vi "DialogCreateInterface.vi"(0 "ClassWriterNative.lvclass":refnum<class "ClassWriterNative.lvclass">, 1 "ProjectItem Refnum":refnum<vi>, 5 "error in (no error)":errorcluster) -> (14 "Reference out":refnum<class "ClassWriterNative.lvclass">, 15 "Cancelled":bool, 16 "CreateInterfaceData":T3, 19 "error out":errorcluster)   [LabVIEW 2020, in "ClassWriterNative.lvclass"]
uses:
  <resource>/Framework/Providers/Open_GDS/ClassProviders/Provider_LvNativeClass/ClassWriterNative_class/ClassWriterNative.lvclass
  <resource>/Framework/Providers/Open_GDS/ClassProviders/Provider_BaseClassInterface/CreateInterfaceData.ctl
  <resource>/Framework/Providers/Open_GDS/ClassProviders/Provider_BaseClassInterface/ClassWriter_class/InterfaceMethodsToCreate.ctl
  <resource>/Framework/Providers/Open_GDS/ClassProviders/Common/CommonVIs/CommonVIs_AttributeType.ctl
  <resource>/Framework/Providers/Open_GDS/ClassProviders/Common/CommonVIs/CommonVIs_AttributeDataType.ctl
  <resource>/Framework/Providers/Open_GDS/ClassProviders/Common/String/GDSString_AccessScopeModifierType.ctl
  <resource>/Framework/Providers/Open_GDS/ClassProviders/Provider_BaseClassInterface/ClassWriter_class/InterfacesToImplement.ctl
  <resource>/Framework/Providers/Open_GDS/ClassProviders/Provider_BaseClassInterface/BaseProvider_SubVIs/BaseProvider_WireList.ctl
  <resource>/Framework/Providers/Open_GDS/ClassProviders/Provider_BaseClassInterface/BaseProvider_SubVIs/BaseProvider_WireStyleType.ctl
  <vilib>/Utility/miscctls.llb/LVRectTypeDef.ctl
  <resource>/Framework/Providers/Open_GDS/ClassProviders/Common/InterfaceLibrary/InterfaceInfo.ctl
  <resource>/Framework/Providers/Open_GDS/ClassProviders/Common/LvClass_class/GDSLvClass_ClassMethodInfo.ctl
  <resource>/Framework/Providers/Open_GDS/ClassProviders/Common/CommonVIs/CommonVIs_ClassIconSelection_Action.ctl
  <vilib>/Utility/miscctls.llb/LVPositionTypeDef.ctl
  <vilib>/picture/picture.llb/imagedata.ctl
  <vilib>/Utility/miscctls.llb/LVRowAndColumnUnsignedTypeDef.ctl
  8226ef7b-d77c-4b82-be33-8974597c5039.vi
  <resource>/Framework/Providers/Open_GDS/ClassProviders/Common/InterfaceLibrary/InterfaceLibrary.lvlib
  <resource>/Framework/Providers/Open_GDS/ClassProviders/Provider_BaseClassInterface/ClassWriter_class/ClassWriter.lvclass
panel:
  out "IconSelection":picture
  in  "WireSelectionList":T1
  out "Wire Style":cluster{"Name":string, "Wire":picture}
  in  "InterfaceFilter":string caption="Filter"
  out "Icon":picture
  in  "_ShowContextHelp":bool
  in  "Help":bool
  in  "ConnectorPanePattern":u16(ring) caption="Connector Pane" items=["4x4x4", "5x6x5", "6x8x6"]
  in  "_UseLLB":bool
  in  "_InterfaceFolderSuffix":string caption="Interface Folder Suffix"
  out "ProductPicture":picture
  out "DupPath":bool
  in  "_InterfaceName":string caption="Interface Name"
  in  "_ClassDescription":string caption="Interface Description"
  in  "_InterfaceFolder":path caption="Save Interface To.."
  out "TriggerSuffixChange":string
  in  "SelectInterfaceClass":i32[](listbox) caption="Select Parent Interface(s) (ctrl+click to do multiple Selection)"
  in  "Methods":string[][](table) caption="3 methods selected"
  in  "Cancel":bool
  in  "CreateInterface":bool
  # "Icon"
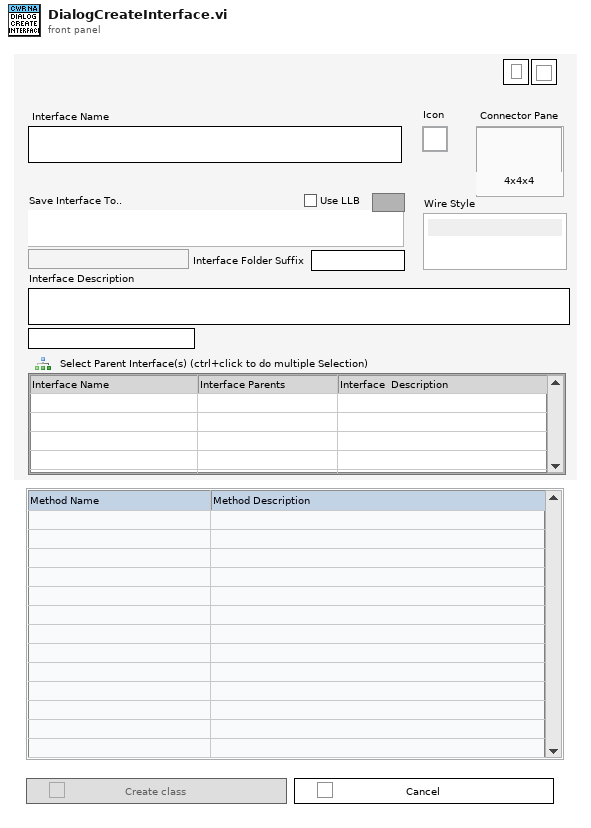
[diagram p1: front panel]
types:
  T1 = typedef "BaseProvider_WireList.ctl" = cluster{"WireStyle":T2[], "WireEditor":bool}
  T2 = typedef "BaseProvider_WireStyleType.ctl" = cluster{"Boolean":bool, "Wire":picture, "Name":string, "Status":u16}
  T3 = typedef "ClassWriter.lvclass/CreateInterfaceData.ctl" = cluster{"InterfaceName":string, "InterfaceFolder":path, "InterfaceDescription":string, "FolderSuffix":string, "MethodsToCreate":T4[], "ParentInterfaces":T8}
  T4 = typedef "ClassWriter.lvclass/InterfaceMethodsToCreate.ctl" = cluster{"Name":string, "Description":string, "MethodsArgumentsIn":T5[], "MethodsArgumentsOut":T5[]}
  T5 = typedef "CommonVIs_AttributeType.ctl" = cluster{"Name":string, "DataType":T6, "ArrayDim":i32, "CtrlPath":path, "DataTypeString":string, "AccessScope":T7, "InitialData":variant}
  T6 = typedef "CommonVIs_AttributeDataType.ctl" = enum16{"UINT8", "INT8", "UINT16", "INT16", "UINT32", "INT32", "UINT64", "INT64", "SGL", "DBL", "EXT", "CSG", "CDB", "CXT", "TimeStamp", "STRING", "PATH", "BOOL", "ENUM", "RefNum", "VIRefNum", "LabVIEW Class", "Cluster", "Variant", "TypeDef", "Waveform", "LabVIEW Object", "Other", "void"}
  T7 = typedef "GDSString_AccessScopeModifierType.ctl" = enum16{"public", "private", "protected", "internal"}
  T8 = typedef "ClassWriter.lvclass/InterfacesToImplement.ctl" = cluster{"InterfacePath":path[], "CreateMethods":bool, "MethodsPerInterface(Empty=>All)":cluster{"Methods":string[]}[]}
  T9 = typedef "LVPositionTypeDef.ctl" = cluster{"Left":i32, "Top":i32}
  T10 = cluster{"Font Name":string, "Size":u16, "Bold":bool, "Italic":bool, "Underline":bool, "Strikeout":bool, "Color":u32}
  T11 = typedef "CommonVIs_ClassIconSelection_Action.ctl" = enum16{"All", "Non Interface", "Only Interface"}
  T12 = typedef "LVRectTypeDef.ctl" = cluster{"Left":i16, "Top":i16, "Right":i16, "Bottom":i16}
  T13 = typedef "InterfaceLibrary.lvlib/InterfaceInfo.ctl" = cluster{"Name(Short if no Conflicts)":string, "FullQualifierName":string, "Description":string, "Path":path, "ParentInterfaceNames(Short if no Conflitcs)":string[], "ParentInterfaceFullQualifierNames":string[], "IconPath":path, "Methods":T14[], "DynamicDispatchMethod":bool[]}
  T14 = typedef "GDSLvClass_ClassMethodInfo.ctl" = cluster{"Name":string, "Descriptions":string, "RelativePath":path, "SourceScope":enum32{"invalid scope", "public", "private", "protected", "community"}, "MustOverride":bool, "VirtualFolderLocation":string[]}
  T15 = cluster{"Cancel":bool, "Derived":bool, "DeriveFromClassRef":refnum<vi>, "ClassPaths":path[], "DesignPatternsVisible":bool, "ClassProviderName":string, "InitDerived":bool, "ClassFolderSuffix":string, "LLB_Allowed":bool, "StartFolder":path, "SplitterMouseDown":bool, "OldBnds":T12, "BondsChanged":bool, "StartBnds":T12, "InterfaceInfo":T13[], "InterfaceIcons":path[]}
  T16 = typedef "LVPointTypeDef.ctl" = cluster{"Horizontal":i16, "Vertical":i16}
  T17 = enum8{"Enabled", "Disabled", "Disabled and Grayed Out"}
  T18 = typedef "imagedata.ctl" = cluster{"image type":i32, "image depth":i32, "image":u8[], "mask":u8[], "colors":u32[], "Rectangle":cluster{"left":i16, "top":i16, "right":i16, "bottom":i16}}
  T19 = typedef "LVRowAndColumnUnsignedTypeDef.ctl" = cluster{"Row":u32, "Column":u32}
  T20 = typedef "BaseProvider_IniFileSettings.ctl" = cluster{"ClassFolderSuffix":string, "InterfaceFolderSuffix":string, "InterfaceIcon":string}
  T21 = typedef "Scripting_ConnectorPanePatternType.ctl" = u16
  T22 = enum32{"Invalid", "Standard", "Closed", "Hidden", "Minimized", "Maximized"}
  T23 = typedef "GOOP_WireConfigurationType.ctl" = cluster{"Edge thickness":i32, "Edge color":u32, "Center thickness":i32, "Center pattern":T24, "CenterColor1":u32, "CenterColor2":u32, "Tunnels and terminals colors":u32}
  T24 = typedef "GOOP_WirePattern.ctl" = enum16{"Solid", "Large dash", "Small dash"}
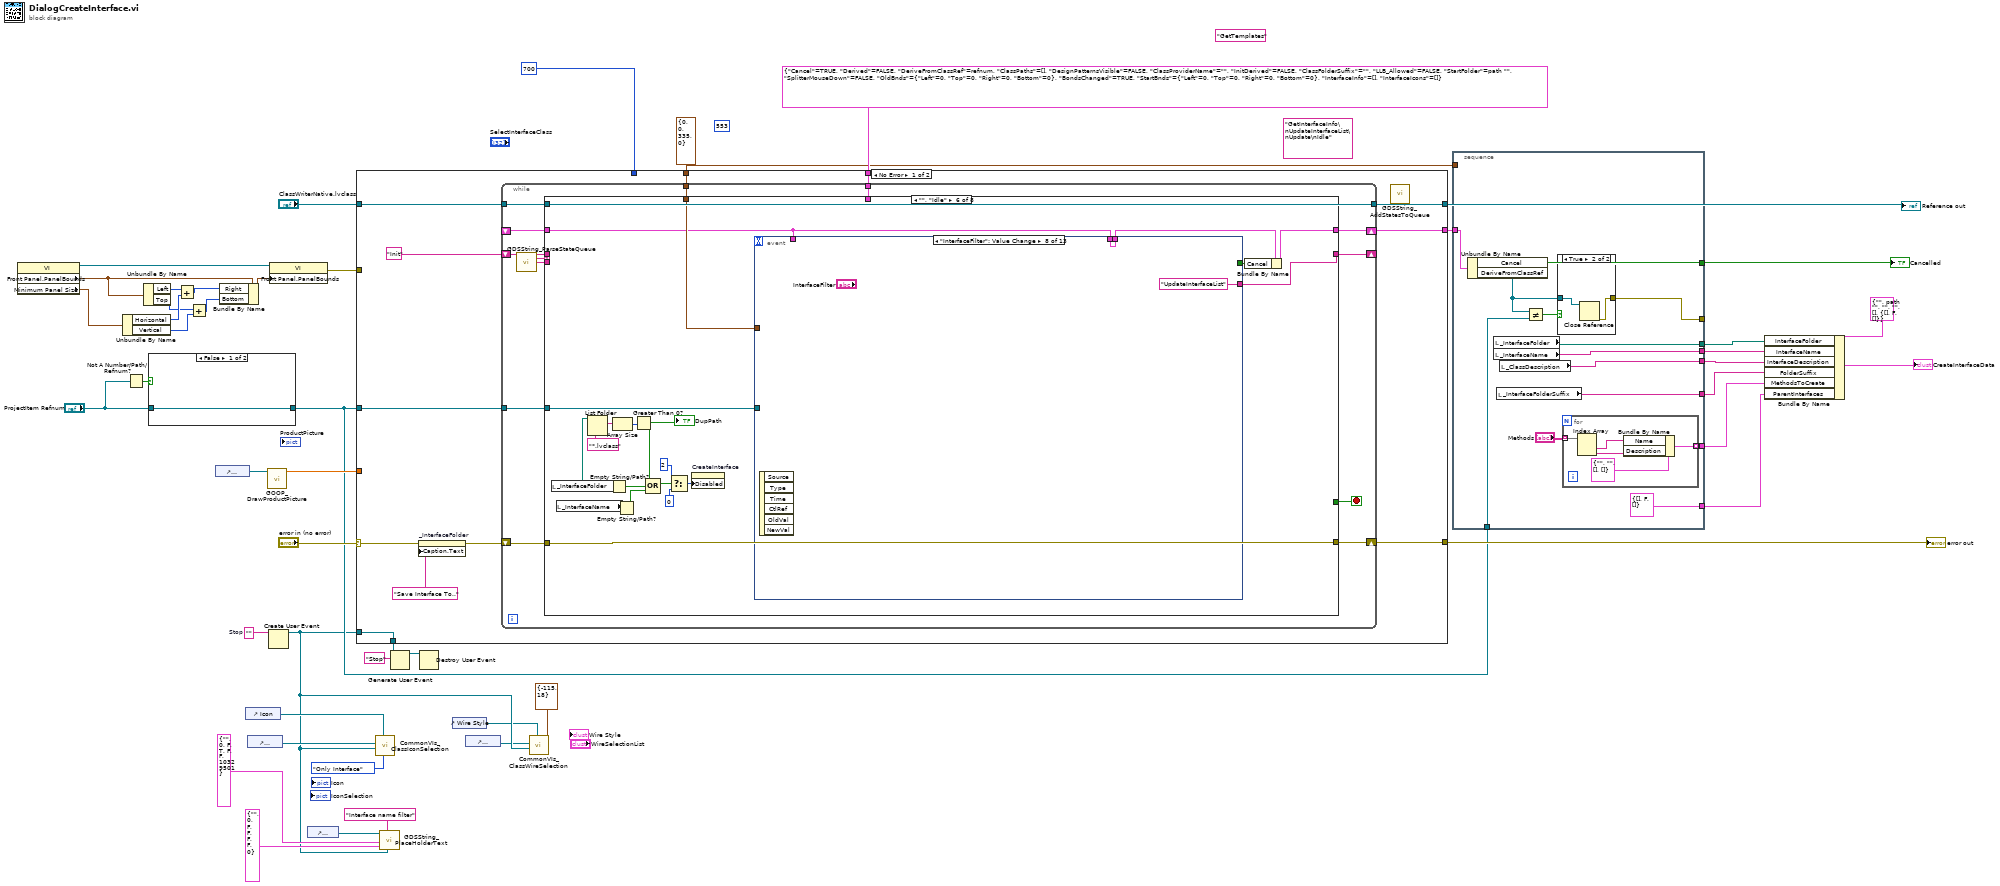
[diagram p0: block diagram]
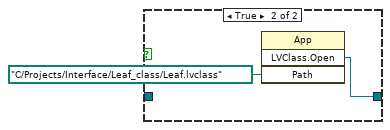
[diagram p2: hidden frame]
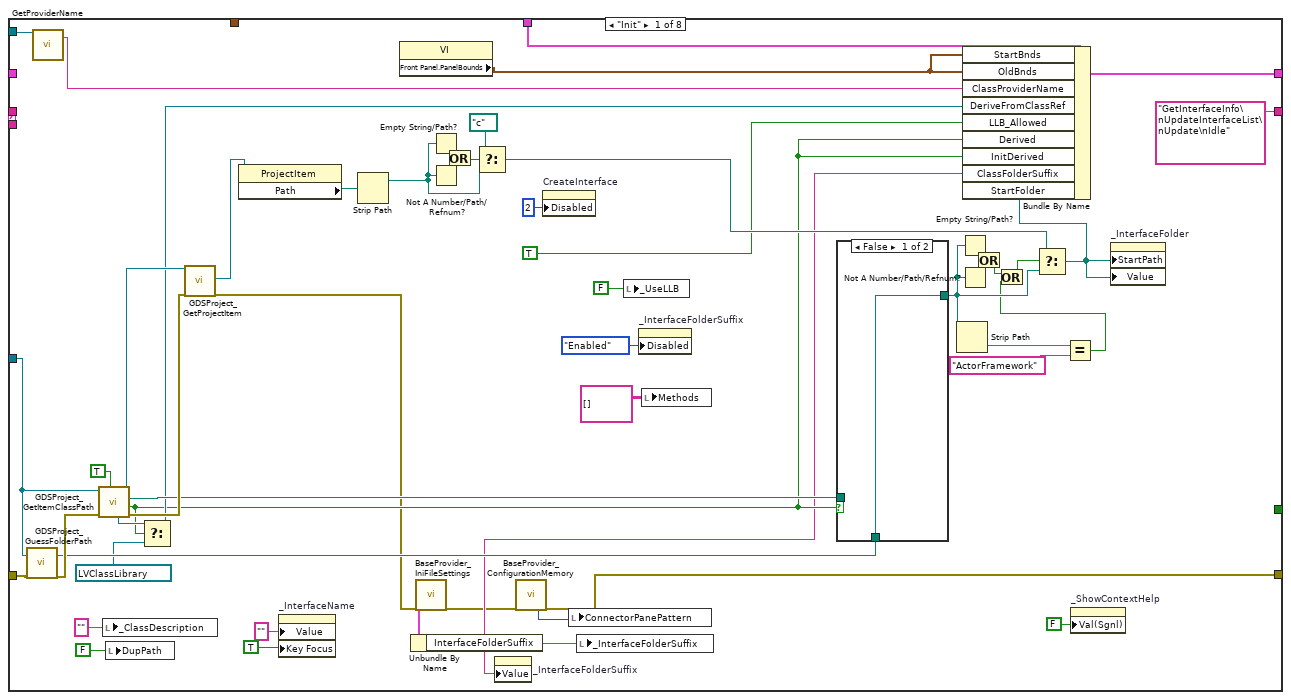
[diagram p4: hidden frame]
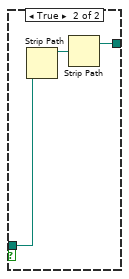
[diagram p5: hidden frame]
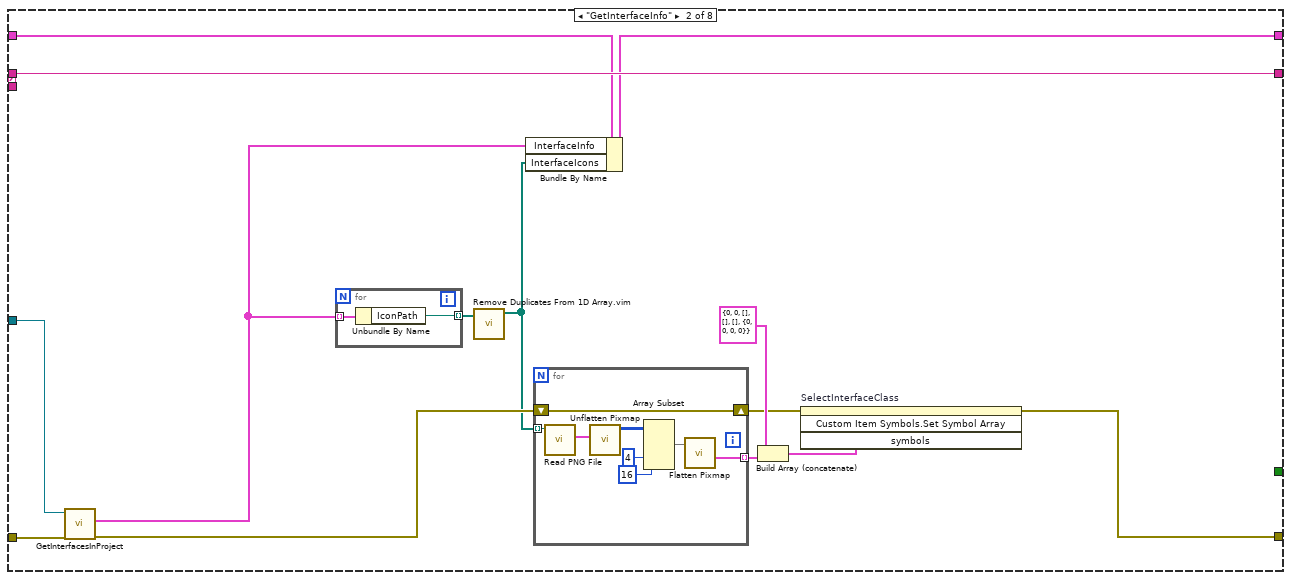
[diagram p6: hidden frame]
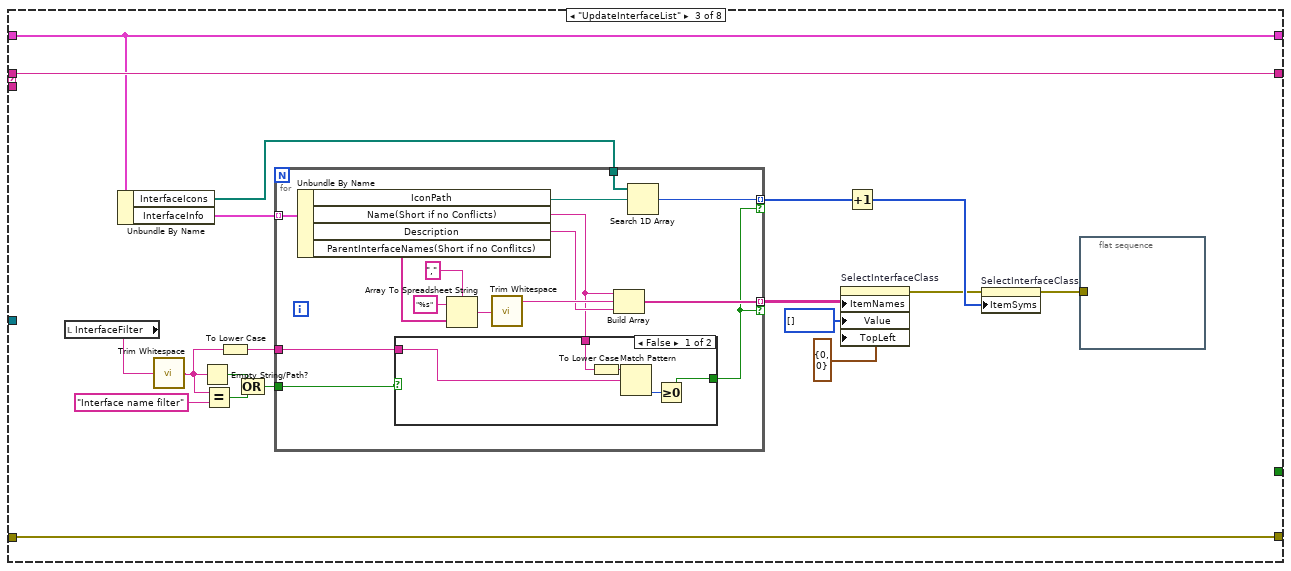
[diagram p7: hidden frame]
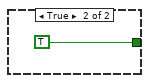
[diagram p8: hidden frame]
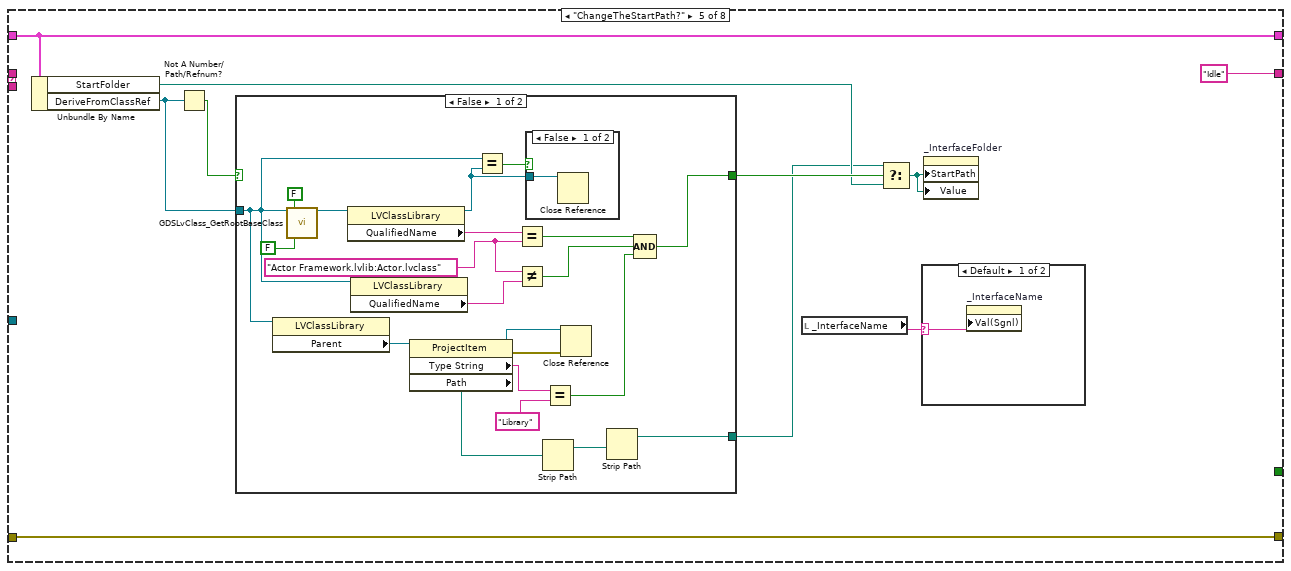
[diagram p10: hidden frame]
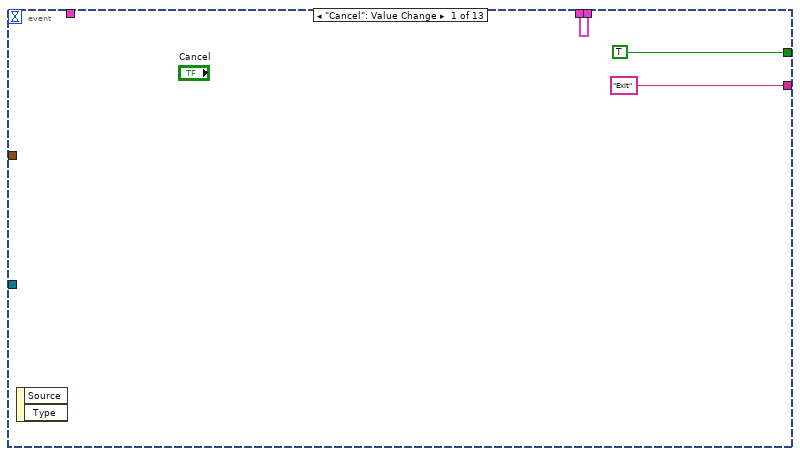
[diagram p14: hidden frame]
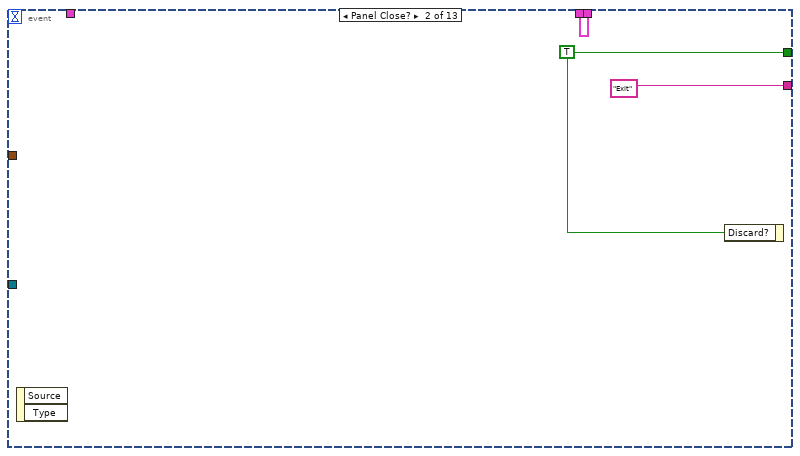
[diagram p15: hidden frame]
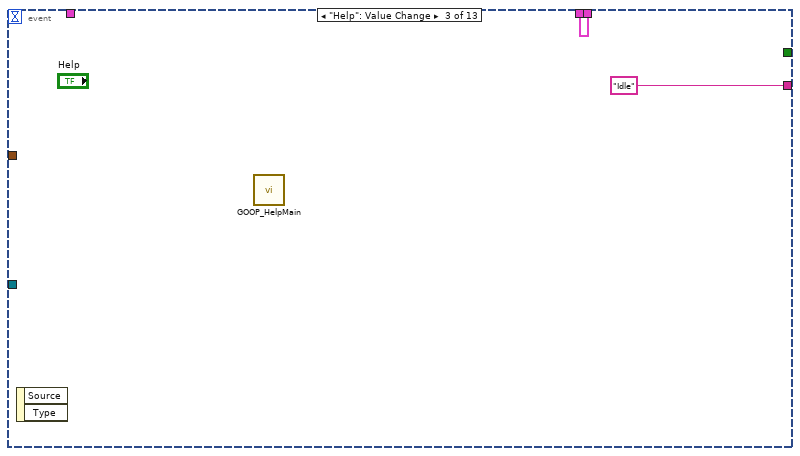
[diagram p16: hidden frame]
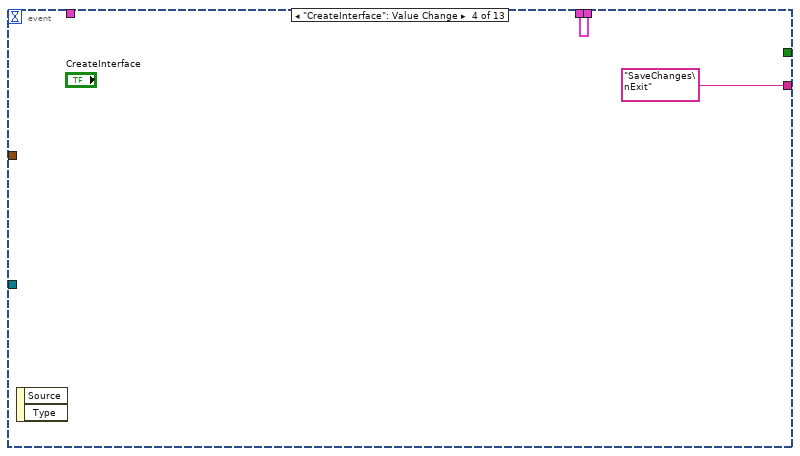
[diagram p17: hidden frame]
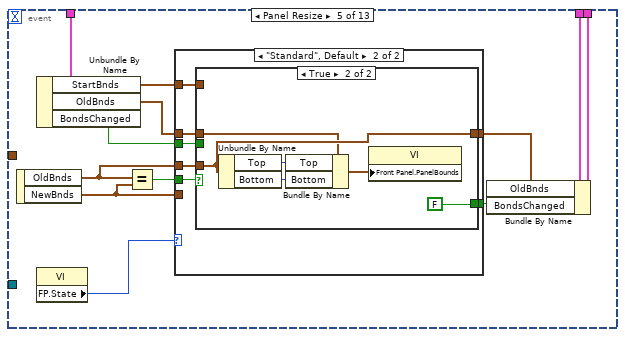
[diagram p18: hidden frame]
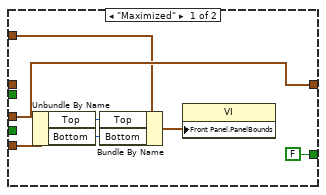
[diagram p19: hidden frame]
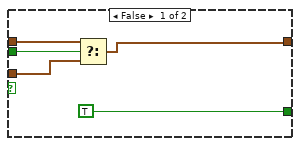
[diagram p20: hidden frame]
diagram:
  w6 = ""  # Stop
  (unwired) "GetInterfaceInfo\nUpdateInterfaceList\nUpdate\nIdle"
  (unwired) i16 553 ("Right")
  w38 = T12 {"Left"=0, "Top"=0, "Right"=335, "Bottom"=0} ("Rect")
  (unwired) "GetTemplates"
  n1 = property class="VI"() -> (reference out=w34:refnum<vi>, "Front Panel.PanelBounds"=w32:T12, "Minimum Panel Size"=w30:T16)  [unwired: 2 in, 1 out]
  n2 = Unbundle By Name(w30) -> ("Horizontal"=w29:i16, "Vertical"=w26:i16)
  n3 = Not A Number/Path/Refnum?(number/path/refnum="ProjectItem Refnum") -> (NaN/Path/Refnum?=w18:bool)
  n4 = Unbundle By Name(w32) -> ("Left"=w31:i16, "Top"=w27:i16)
  n5 = case shown="False" w18 {
    tunnel: "ProjectItem Refnum" -> [w49 _]
    tunnel: [w49 w50] -> w16
    frame False {
    }
    frame True {
      n6 = invoke class="App" method="LVClass.Open"("Path"=path "C:/Projects/Interface/Leaf_class/Leaf.lvclass") -> ("LVClass.Open"=w50:refnum<vi>)  [unwired: 3 in, 3 out]
    }
  }
  n7 = Add(x=w31, y=w29) -> (x+y=w28:i16)
  n8 = Add(x=w27, y=w26) -> (x+y=w25:i16)
  n9 = control-ref of="ProductPicture"() -> (w36:refnum<vi>)
  n10 = Bundle By Name(cluster=w32, "Right"=w28, "Bottom"=w25) -> (w33:T12)
  n11 = control-ref of="Icon"() -> (w22:refnum<vi>)
  n12 = control-ref of="IconSelection"() -> (w21:refnum<vi>)
  n13 = call <resource>:"GOOP_DrawProductPicture.vi"("ProductPictureControl"=w36) -> ("Zoom Factor"=w35:sgl)  [unwired: 10 in]
  n14 = Create User Event(user event datatype=w6) -> (user event=w3:refnum<user-event>)  [unwired: 1 in, 1 out]
  n15 = property class="VI"(reference=w34, "Front Panel.PanelBounds"=w33) -> (error out=w24:errorcluster)  [unwired: 1 in, 1 out]
  n16 = control-ref of="InterfaceFilter"() -> (w7:refnum<vi>)
  n17 = case shown="No Error" "error in (no error)" {
    selector: "error in (no error)" -> [w55 w387]
    tunnel: "ClassWriterNative.lvclass" -> [w61 w386]
    tunnel: [w53 w387] -> w47
    tunnel: [w62 w386] -> w45
    tunnel: T15 {"Cancel"=TRUE, "Derived"=FALSE, "DeriveFromClassRef"=refnum, "ClassPaths"=[], "DesignPatternsVisible"=FALSE, "ClassProviderName"="", "InitDerived"=FALSE, "ClassFolderSuffix"="", "LLB_Allowed"=FALSE, "StartFolder"=path "", "SplitterMouseDown"=FALSE, "OldBnds"={"Left"=0, "Top"=0, "Right"=0, "Bottom"=0}, "BondsChanged"=TRUE, "StartBnds"={"Left"=0, "Top"=0, "Right"=0, "Bottom"=0}, "InterfaceInfo"=[], "InterfaceIcons"=[]} ("output cluster") -> [w60 _]
    tunnel: w16 -> [w59 _]
    tunnel: [w58 _] -> w43
    tunnel: w38 -> [w57 _]
    tunnel: w35 -> [_ _]
    tunnel: w24 -> [_ _]
    tunnel: [w52 w385] -> w19
    tunnel: w3 -> [w52 w385]
    tunnel: 700 ("Splitter Position") -> [_ _]
    frame No Error {
      n18 = property on="_InterfaceFolder" class="Path"(error in=w55, "Caption.Text"="Save Interface To.." ("t")) -> (error out=w56:errorcluster)  [unwired: 1 in, 1 out]
      n19 = while {
        shift-right: [w75] -> w53
        shift-left: w56 -> [w77]
        shift-right: [w65] -> _
        shift-left: "Init" -> [w69]
        shift-right: [w71] -> w58
        shift-left: _ -> [w76]
        tunnel: w61 -> [w74]
        tunnel: [w74] -> w62
        tunnel: w60 -> [w73]
        tunnel: w59 -> [w72]
        tunnel: w57 -> [w70]
        stop <- w64 stop-if-true
        n20 = call <resource>:"GDSString_ParseStateQueue.vi"("State Queue"=w69) -> ("Remaining States"=w67:string, "Current State"=w68:string, "Arguments"=w66:string)  [unwired: 10 in, 2 out]
        n21 = case shown="\"\", \"Idle\"" w68 {
          tunnel: w76 -> [_ w144 w156 w198 w207 w232 w378 w384]
          tunnel: [w126 w141 w156 w198 w207 w248 w378 w384] -> w71
          tunnel: w77 -> [w109 w143 w174 w196 w203 w251 w377 w381]
          tunnel: [w81 w134 w174 w196 w203 w251 w377 w381] -> w75
          tunnel: w74 -> [w103 _ _ _ _ _ _ _]
          tunnel: ["GetInterfaceInfo\nUpdateInterfaceList\nUpdate\nIdle" w145 w173 w197 "Idle" w249 w376 "Exit"] -> w65
          tunnel: w73 -> [w125 _ _ _ _ _ _ _]
          tunnel: w72 -> [w107 w142 _ _ _ w235 _ _]
          tunnel: w70 -> [_ _ _ _ _ w233 _ _]
          tunnel: w67 -> [_ w145 w173 w197 _ _ w376 _]
          tunnel: w66 -> [_ _ _ _ _ _ _ _]
          tunnel: [_ _ _ _ _ _ _ TRUE] -> w64
          frame "Init" {
            n22 = call <resource>:"GDSProject_GuessFolderPath.vi"("ProjectItem"=w107, "error in (no error)"=w109) -> ("Path"=w106:path, "error out"=w108:errorcluster)  [unwired: 14 in, 2 out]
            n23 = call-dynamic "GetProviderName.vi"("ClassWriterNative in"=w103) -> ("ProviderName"=w95:string)  [unwired: 16 in, 2 out]
            n24 = call <resource>:"GDSProject_GetItemClassPath.vi"("ReturnRefToClass(False)"=TRUE, "error in"=w108, "ProjectItemRefIn"=w107) -> ("error out"=w123:errorcluster, "LvCLassFound"=w97:bool, "Path"=w104:path, "ProjectItemRefOut"=w122:refnum<vi>, "LvClassRef"=w100:refnum<vi>)  [unwired: 3 in, 1 out]
            n25 = local write "_ClassDescription"("" ("Class description")) -> ()
            n26 = local write "DupPath"(FALSE ("DupPath")) -> ()
            n27 = Select(t=w100, s=w97, f=refnum<vi> refnum) -> (s? t:f=w99:refnum<vi>)
            n28 = call <resource>:"GDSProject_GetProjectItem.vi"("ProjectItemToSearchFrom"=w122, "error in (no error)"=w123) -> ("ProjectItemFound"=w116:refnum<vi>, "error out"=w82:errorcluster)  [unwired: 14 in, 2 out]
            n29 = property class="ProjectItem"(reference=w116) -> ("Path"=w111:path)  [unwired: 1 in, 2 out]
            n30 = property on="_InterfaceName" class="Str"("Value"="" ("Class name"), "Key Focus"=TRUE) -> ()  [unwired: 2 in, 2 out]
            n31 = Strip Path(path=w111) -> (stripped path=w110:path)  [unwired: 1 out]
            n32 = property class="VI"() -> ("Front Panel.PanelBounds"=w78:T12)  [unwired: 2 in, 2 out]
            n33 = call <resource>:"BaseProvider_IniFileSettings.vi"("error in (no error)"=w82) -> ("IniFileSettings"=w96:T20)  [unwired: 17 in, 1 out]
            n34 = Unbundle By Name(w96) -> ("InterfaceFolderSuffix"=w94:string)
            n35 = Empty String/Path?(string/path=w110) -> (empty?=w112:bool)
            n36 = Not A Number/Path/Refnum?(number/path/refnum=w110) -> (NaN/Path/Refnum?=w113:bool)
            n37 = Or(x=w112, y=w113) -> (x .or. y?=w114:bool)
            n38 = Select(t=path "c:/", s=w114, f=w110) -> (s? t:f=w101:path)
            n39 = property on="_InterfaceFolderSuffix" class="Str"("Value"=w94) -> ()  [unwired: 2 in, 2 out]
            n40 = call <resource>:"BaseProvider_ConfigurationMemory.vi"("error in (no error)"=w82) -> ("PatternOut"=w80:T21, "error out"=w81:errorcluster)  [unwired: 12 in, 5 out]
            n41 = property on="CreateInterface" class="Bool"("Disabled"=u8 2) -> ()  [unwired: 2 in, 2 out]
            n42 = local write "ConnectorPanePattern"(w80) -> ()
            n43 = local write "_InterfaceFolderSuffix"(w94) -> ()
            n44 = local write "_UseLLB"(FALSE ("_UseLLB")) -> ()
            n45 = property on="_InterfaceFolderSuffix" class="Str"("Disabled"=T17."Enabled") -> ()  [unwired: 2 in, 2 out]
            n46 = local write "Methods"(string[][] [] ("Methods")) -> ()
            n47 = case shown="False" w97 {
              tunnel: w104 -> [_ w131]
              tunnel: [w128 w129] -> w92
              tunnel: w106 -> [w128 _]
              frame False {
              }
              frame True {
                n48 = Strip Path(path=w131) -> (stripped path=w130:path)  [unwired: 1 out]
                n49 = Strip Path(path=w130) -> (stripped path=w129:path)  [unwired: 1 out]
              }
            }
            n50 = Strip Path(path=w92) -> (name=w91:string)  [unwired: 1 out]
            n51 = Empty String/Path?(string/path=w92) -> (empty?=w118:bool)
            n52 = Not A Number/Path/Refnum?(number/path/refnum=w92) -> (NaN/Path/Refnum?=w117:bool)
            n53 = Or(x=w118, y=w117) -> (x .or. y?=w89:bool)
            n54 = Equal?(x=w91, y="ActorFramework") -> (x = y?=w88:bool)
            n55 = Or(x=w89, y=w88) -> (x .or. y?=w87:bool)
            n56 = Select(t=w101, s=w87, f=w92) -> (s? t:f=w93:path)
            n57 = Bundle By Name(cluster=w125, "StartBnds"=w78, "OldBnds"=w78, "ClassProviderName"=w95, "DeriveFromClassRef"=w99, "LLB_Allowed"=TRUE, "Derived"=w97, "InitDerived"=w97, "ClassFolderSuffix"=w94, "StartFolder"=w93) -> (w126:T15)
            n58 = property on="_ShowContextHelp" class="Bool (strict)"("Val(Sgnl)"=FALSE ("Value (Signaling)")) -> ()  [unwired: 2 in, 2 out]
            n59 = property on="_InterfaceFolder" class="Path"("StartPath"=w93, "Value"=w93) -> ()  [unwired: 2 in, 2 out]
          }
          frame "GetInterfaceInfo" {
            n60 = call <resource>:"GetInterfacesInProject.vi"("error in"=w143, "Project/ProjectItem"=w142) -> ("error out"=w135:errorcluster, "InterfaceInfo"=w133:T13[])  [unwired: 8 in]
            n61 = for {
              tunnel: w133 -> [w155] mode=indexing
              tunnel: [w154] -> w136 mode=indexing
              n62 = Unbundle By Name(w155) -> ("IconPath"=w154:path)
            }
            n63 = call "Remove Duplicates From 1D Array.vim"("array"=w136) -> ("array with duplicates removed"=w132:path[])  [unwired: 10 in]
            n64 = Bundle By Name(cluster=w144, "InterfaceInfo"=w133, "InterfaceIcons"=w132) -> (w141:T15)
            n65 = for {
              tunnel: w132 -> [w153] mode=indexing
              shift-right: [w147] -> w137
              shift-left: w135 -> [w147]
              tunnel: [w146] -> w138 mode=indexing
              n66 = call <vilib>:"Read PNG File.vi"("path to PNG file"=w153) -> ("image data"=w152:T18)  [unwired: 8 in, 2 out]
              n67 = call <vilib>:"Unflatten Pixmap.vi"("image data"=w152) -> ("24-bit pixmap"=w151:u32[][])  [unwired: 4 in, 6 out]
              n68 = Array Subset(array=w151, index (col)=4 ("index"), length (col)=16 ("length")) -> (w148:u32[][])  [unwired: 2 in]
              n69 = call <vilib>:"Flatten Pixmap.vi"("24-bit pixmap"=w148) -> ("image data"=w146:T18)  [unwired: 10 in]
            }
            n70 = Build Array (concatenate)(T18 {"image type"=0, "image depth"=0, "image"=[], "mask"=[], "colors"=[], "Rectangle"={"left"=0, "top"=0, "right"=0, "bottom"=0}} ("image data"), w138) -> (w140:T18[])
            n71 = invoke on="SelectInterfaceClass" class="MCListbox (strict)" method="Custom Item Symbols.Set Symbol Array"(error in=w137, "symbols"=w140) -> (error out=w134:errorcluster)  [unwired: 2 in, 3 out]
          }
          frame "UpdateInterfaceList" {
            n72 = local read "InterfaceFilter"() -> (w157:string)
            n73 = Unbundle By Name(w156) -> ("InterfaceIcons"=w159:path[], "InterfaceInfo"=w158:T13[])
            n74 = call <vilib>:"Trim Whitespace.vi"("string"=w157) -> ("trimmed string"=w166:string)  [unwired: 1 in]
            n75 = Empty String/Path?(string/path=w166) -> (empty?=w163:bool)
            n76 = Equal?(x=w166, y="Interface name filter" ("InterfaceFilter")) -> (x = y?=w164:bool)
            n77 = To Lower Case(string=w166) -> (all lower case string=w170:string)
            n78 = Compound Arithmetic op=OR(w163, w164) -> (w165:bool)
            n79 = for {
              tunnel: [w185] -> w160 mode=indexing if=w177
              tunnel: w158 -> [w184] mode=indexing
              tunnel: w159 -> [w180]
              tunnel: [w179] -> w171 mode=indexing if=w177
              tunnel: w165 -> [w178]
              tunnel: w170 -> [w175]
              n80 = Unbundle By Name(w184) -> ("IconPath"=w181:path, "Name(Short if no Conflicts)"=w176:string, "Description"=w182:string, "ParentInterfaceNames(Short if no Conflitcs)"=w183:string[])
              n81 = case shown="False" w178 {
                tunnel: [w191 TRUE] -> w177
                tunnel: w176 -> [w194 _]
                tunnel: w175 -> [w193 _]
                frame False {
                  n82 = To Lower Case(string=w194) -> (all lower case string=w190:string)
                  n83 = Match Pattern(string=w190, regular expression=w193) -> (offset past match=w192:i32)  [unwired: 1 in, 3 out]
                  n84 = Greater Or Equal To 0?(x=w192) -> (x >= 0?=w191:bool)
                }
                frame True {
                }
              }
              n85 = Array To Spreadsheet String(delimiter (Tab)=",", array=w183, 3:"%s" ("format string")) -> (spreadsheet string=w187:string)
              n86 = call <vilib>:"Trim Whitespace.vi"("string"=w187) -> ("trimmed string"=w186:string)  [unwired: 1 in]
              n87 = Build Array(w176, w186, w182) -> (w185:string[])
              n88 = Search 1D Array(1D array=w180, element=w181) -> (index of element=w179:i32)  [unwired: 1 in]
            }
            n89 = property on="SelectInterfaceClass" class="MCListbox (strict)"("ItemNames"=w160, "Value"=i32[] [] ("_SelectInterfaceClass"), "TopLeft"=T19 {"Row"=0, "Column"=0} ("Top Left Visible Cell")) -> (error out=w161:errorcluster)  [unwired: 2 in, 1 out]
            n90 = Increment(x=w171) -> (x+1=w172:i32[])
            n91 = property on="SelectInterfaceClass" class="MCListbox (strict)"(error in=w161, "ItemSyms"=w172) -> (error out=w169:errorcluster)  [unwired: 1 in, 1 out]
            n92 = flat-sequence {
              tunnel: w169 -> [_]
              frame #0 {
              }
            }
          }
          frame "Update" {
          }
          frame "ChangeTheStartPath?" {
            n93 = Unbundle By Name(w207) -> ("StartFolder"=w201:path, "DeriveFromClassRef"=w205:refnum<vi>)
            n94 = Not A Number/Path/Refnum?(number/path/refnum=w205) -> (NaN/Path/Refnum?=w202:bool)
            n95 = case shown="False" w202 {
              tunnel: w205 -> [w213 _]
              tunnel: [w214 _] -> w204
              tunnel: [w217 _] -> w200
              frame False {
                w211 = "Actor Framework.lvlib:Actor.lvclass" ("y")
                n96 = property class="LVClassLibrary"(reference=w213) -> ("Parent"=w224:refnum<vi>)  [unwired: 1 in, 2 out]
                n97 = call <resource>:"GDSLvClass_GetRootBaseClass.vi"("ViRef/Path,LvClassRef/Path"=w213, "Don'tOpenReference"=FALSE, "LimitToSpecificProviderTypeOfSameType(True)"=FALSE) -> ("RootBaseClassRef"=w225:refnum<vi>)  [unwired: 11 in, 5 out]
                n98 = property class="LVClassLibrary"(reference=w225) -> (reference out=w226:refnum<vi>, "QualifiedName"=w228:string)  [unwired: 1 in, 1 out]
                n99 = property class="LVClassLibrary"(reference=w213) -> ("QualifiedName"=w212:string)  [unwired: 1 in, 2 out]
                n100 = property class="ProjectItem"(reference=w224) -> (reference out=w220:refnum<vi>, error out=w221:errorcluster, "Type String"=w223:string, "Path"=w219:path)  [unwired: 1 in]
                n101 = Equal?(x=w213, y=w226) -> (x = y?=w227:bool)
                n102 = Equal?(x=w228, y=w211) -> (x = y?=w216:bool)
                n103 = Not Equal?(x=w211, y=w212) -> (x != y?=w210:bool)
                n104 = case shown="False" w227 {
                  tunnel: w226 -> [w231 _]
                  frame False {
                    n105 = Close Reference(reference=w231) -> ()  [unwired: 1 in, 1 out]
                  }
                  frame True {
                  }
                }
                n106 = Strip Path(path=w219) -> (stripped path=w218:path)  [unwired: 1 out]
                n107 = Equal?(x=w223, y="Library") -> (x = y?=w215:bool)
                n108 = Close Reference(reference=w220, error in (no error)=w221) -> ()  [unwired: 1 out]
                n109 = Strip Path(path=w218) -> (stripped path=w217:path)  [unwired: 1 out]
                n110 = Compound Arithmetic op=AND(w216, w210, w215) -> (w214:bool)
              }
              frame True {
              }
            }
            n111 = local read "_InterfaceName"() -> (w199:string)
            n112 = Select(t=w200, s=w204, f=w201) -> (s? t:f=w206:path)
            n113 = case shown="Default" w199 {
              selector: w199 -> [w209 _]
              frame Default {
                n114 = property on="_InterfaceName" class="Str"("Val(Sgnl)"=w209) -> ()  [unwired: 2 in, 2 out]
              }
              frame "" {
              }
            }
            n115 = property on="_InterfaceFolder" class="Path"("StartPath"=w206, "Value"=w206) -> ()  [unwired: 2 in, 2 out]
          }
          frame "", "Idle" {
            n116 = local read "_InterfaceFolder"() -> (w240:path)
            n117 = local read "_InterfaceName"() -> (w241:string)
            n118 = List Folder(path=w240, pattern="*.lvclass") -> (filenames=w238:string[])  [unwired: 2 in, 3 out]
            n119 = Empty String/Path?(string/path=w240) -> (empty?=w243:bool)
            n120 = Array Size(array=w238) -> (size(s)=w237:i32)
            n121 = Empty String/Path?(string/path=w241) -> (empty?=w242:bool)
            n122 = Greater Than 0?(x=w237) -> (x > 0?=w236:bool)
            "DupPath" <- w236
            n123 = Compound Arithmetic op=OR(w236, w243, w242) -> (w244:bool)
            n124 = Select(t=u8 2, s=w244, f=u8 0 ("Disabled")) -> (s? t:f=w247:u8)
            n125 = property on="CreateInterface" class="Bool"("Disabled"=w247) -> ()  [unwired: 2 in, 2 out]
            n126 = event shown="[7] \"InterfaceFilter\": Value Change" {
              selector: _ -> [_ _ _ _ _ _ _ _ _ _ _ _ _]
              dyn-events: _ -> [_ _ _ _ _ _ _ _ _ _ _ _ _]
              timeout: _ -> [_ _ _ _ _ _ _ _ _ _ _ _ _]
              tunnel: ["Exit" "Exit" "Idle" "SaveChanges\nExit" _ _ "Idle" "UpdateInterfaceList" "Idle" "Idle" "Idle" "Idle" "Idle"] -> w249
              tunnel: [TRUE w256 _ _ _ _ _ _ _ _ _ _ _] -> w250
              tunnel: w232 -> [_ _ _ _ w268 _ _ _ _ _ _ _ _]
              tunnel: w235 -> [_ _ _ _ _ _ _ _ _ _ _ _ _]
              tunnel: w232 -> [w252 w255 w258 w260 w267 w303 w304 w307 w309 w335 w343 w358 w368]
              tunnel: [w252 w255 w258 w260 w266 w303 w304 w307 w309 w335 w343 w358 w368] -> w234
              tunnel: w233 -> [_ _ _ _ _ _ _ _ _ _ _ _ _]
              event "Cancel": Value Change {
                n127 = event-data() -> ()  [unwired: 1 in, 2 out]
              }
              event Panel Close? {
                w256 = TRUE
                n128 = event-data() -> ()  [unwired: 1 in, 2 out]
                n129 = event-data("Discard?"=w256) -> ()  [unwired: 1 in, 1 out]
              }
              event "Help": Value Change {
                n130 = event-data() -> ()  [unwired: 1 in, 2 out]
                n131 = call <resource>:"GOOP_HelpMain.vi"() -> ()  [unwired: 12 in]
              }
              event "CreateInterface": Value Change {
                n132 = event-data() -> ()  [unwired: 1 in, 2 out]
              }
              event Panel Resize {
                n133 = event-data() -> ("OldBnds"=w265:T12, "NewBnds"=w263:T12)  [unwired: 1 in]
                n134 = Unbundle By Name(w268) -> ("StartBnds"=w262:T12, "OldBnds"=w270:T12, "BondsChanged"=w272:bool)
                n135 = property class="VI"() -> ("FP.State"=w264:T22)  [unwired: 2 in, 2 out]
                n136 = Equal?(x=w265, y=w263) -> (x = y?=w269:bool)
                n137 = case shown="\"Standard\", Default" w264 {
                  tunnel: [w275 w287] -> w273
                  tunnel: w272 -> [_ w286]
                  tunnel: [FALSE w285] -> w271
                  tunnel: w270 -> [_ w284]
                  tunnel: w269 -> [_ w283]
                  tunnel: w265 -> [w275 w282]
                  tunnel: w263 -> [w278 _]
                  tunnel: w262 -> [w274 w281]
                  frame "Maximized" {
                    n138 = Unbundle By Name(w278) -> ("Top"=w280:i16, "Bottom"=w279:i16)
                    n139 = Bundle By Name(cluster=w274, "Top"=w280, "Bottom"=w279) -> (w277:T12)
                    n140 = property class="VI"("Front Panel.PanelBounds"=w277) -> ()  [unwired: 2 in, 2 out]
                  }
                  frame "Standard", Default {
                    n141 = case shown="True" w283 {
                      tunnel: w282 -> [w289 w294]
                      tunnel: [w290 w294] -> w287
                      tunnel: w284 -> [w291 w293]
                      tunnel: [TRUE FALSE] -> w285
                      tunnel: w286 -> [w288 _]
                      tunnel: w281 -> [_ _]
                      frame False {
                        n142 = Select(t=w291, s=w288, f=w289) -> (s? t:f=w290:T12)
                      }
                      frame True {
                        n143 = Unbundle By Name(w294) -> ("Top"=w298:i16, "Bottom"=w297:i16)
                        n144 = Bundle By Name(cluster=w293, "Top"=w298, "Bottom"=w297) -> (w296:T12)
                        n145 = property class="VI"("Front Panel.PanelBounds"=w296) -> ()  [unwired: 2 in, 2 out]
                      }
                    }
                  }
                }
                n146 = Bundle By Name(cluster=w267, "OldBnds"=w273, "BondsChanged"=w271) -> (w266:T15)
              }
              event "ConnectorPanePattern": Value Change {
                n147 = event-data() -> ()  [unwired: 1 in, 6 out]
                n148 = call <resource>:"BaseProvider_ConfigurationMemory.vi"() -> ("WireConfigurationOut"=w301:T23, "IconOut"=w302:string)  [unwired: 13 in, 5 out]
                n149 = call <resource>:"BaseProvider_ConfigurationMemory.vi"("WireConfiguration"=w301, "Icon"=w302, "Action"=enum16{"Read", "Load", "Save", "Set"}."Save", "PatternIn"="ConnectorPanePattern") -> ()  [unwired: 9 in, 7 out]
              }
              event "_ClassDescription": Value Change {
                n150 = event-data() -> ()  [unwired: 1 in, 2 out]
              }
              event "InterfaceFilter": Value Change {
                n151 = event-data() -> ()  [unwired: 1 in, 6 out]
              }
              event "_InterfaceName": Value Change {
                n152 = event-data() -> ("OldVal"=w312:string)  [unwired: 1 in]
                n153 = local read "_InterfaceFolder"() -> (w319:path)
                n154 = local read "_InterfaceFolderSuffix"() -> (w308:string)
                n155 = Concatenate Strings(w312, ".llb" ("t")) -> (w310:string)
                n156 = call <resource>:"GOOP300_RemoveUnwantedChars.vi"("StringIn"="_InterfaceName") -> ("StringOut"=w322:string)  [unwired: 10 in]
                n157 = Strip Path(path=w319) -> (stripped path=w320:path, name=w313:string)
                n158 = Concatenate Strings(w312, w308) -> (w321:string)
                n159 = local write "_InterfaceName"(w322) -> ()
                n160 = Equal?(x=w313, y=w321) -> (x = y?=w315:bool)
                n161 = Equal?(x=w313, y=w310) -> (x = y?=w314:bool)
                n162 = Or(x=w315, y=w314) -> (x .or. y?=w316:bool)
                n163 = Select(t=w320, s=w316, f=w319) -> (s? t:f=w318:path)
                n164 = local read "_UseLLB"() -> (w317:bool)
                n165 = case shown="Default" w322 {
                  selector: w322 -> [_ w331]
                  tunnel: [w326 w334] -> w325
                  tunnel: w308 -> [_ w329]
                  tunnel: w318 -> [w326 w332]
                  tunnel: w317 -> [_ w330]
                  frame "" {
                  }
                  frame Default {
                    n166 = Select(t=".llb", s=w330, f=w329) -> (s? t:f=w328:string)
                    n167 = Concatenate Strings(w331, w328) -> (w333:string)
                    n168 = Build Path(base path=w332, name or relative path=w333) -> (appended path=w334:path)
                  }
                }
                n169 = local write "_InterfaceFolder"(w325) -> ()
              }
              event "_UseLLB": Value Change {
                n170 = event-data() -> ()  [unwired: 1 in, 2 out]
                n171 = Select(t=u8 2 ("Disabled"), s="_UseLLB", f=u8 0 ("Disabled")) -> (s? t:f=w339:u8)
                n172 = property on="_InterfaceName" class="Str"() -> ("Value"=w336:string)  [unwired: 2 in, 2 out]
                n173 = property on="_InterfaceFolderSuffix" class="Str"("Disabled"=w339) -> ()  [unwired: 2 in, 2 out]
                n174 = property on="_InterfaceName" class="Str"("Val(Sgnl)"=w336) -> ()  [unwired: 2 in, 2 out]
              }
              event "_ShowContextHelp": Value Change {
                n175 = event-data() -> ("NewVal"=w342:bool)  [unwired: 1 in]
                n176 = Control Help Window(1:w342) -> ()  [unwired: 1 in]
              }
              event "_InterfaceFolderSuffix", "TriggerSuffixChange": Value Change {
                n177 = event-data() -> ("OldVal"=w347:string)  [unwired: 1 in, 2 out]
                n178 = local read "_InterfaceFolder"() -> (w360:path)
                n179 = call <resource>:"GOOP300_RemoveUnwantedChars.vi"("StringIn"="_InterfaceFolderSuffix") -> ("StringOut"=w348:string)  [unwired: 10 in]
                n180 = local write "_InterfaceFolderSuffix"(w348) -> ()
                n181 = Strip Path(path=w360) -> (stripped path=w355:path, name=w357:string)
                n182 = Select(t="", s=FALSE, f=w348) -> (s? t:f=w350:string)
                n183 = Build Array(w348, w347) -> (w346:string[])
                n184 = local read "_InterfaceName"() -> (w352:string)
                n185 = for {
                  tunnel: w346 -> [w362] mode=indexing
                  shift-right: [w363] -> w356
                  shift-left: w357 -> [w366]
                  n186 = Concatenate Strings(w362, "$" ("string")) -> (w365:string)
                  n187 = Match Pattern(string=w366, regular expression=w365) -> (before substring=w363:string)  [unwired: 1 in, 3 out]
                }
                n188 = Empty String/Path?(string/path=w352) -> (empty?=w351:bool)
                n189 = Concatenate Strings(w356, w350) -> (w354:string)
                n190 = Build Path(base path=w355, name or relative path=w354) -> (appended path=w353:path)
                n191 = case shown="False" w351 {
                  tunnel: w353 -> [w367 _]
                  frame False {
                    n192 = local write "_InterfaceFolder"(w367) -> ()
                  }
                  frame True {
                  }
                }
              }
              event "_InterfaceFolder": Value Change {
                n193 = event-data() -> ()  [unwired: 1 in, 2 out]
                n194 = Strip Path(path="_InterfaceFolder") -> ()  [unwired: 2 out]
                n195 = property on="_InterfaceName" class="Str"() -> ("Value"=w369:string)  [unwired: 2 in, 2 out]
                n196 = property on="_InterfaceName" class="Str"("Val(Sgnl)"=w369) -> ()  [unwired: 2 in, 2 out]
              }
            }
            n197 = Bundle By Name(cluster=w234, "Cancel"=w250) -> (w248:T15)
          }
          frame "SaveChanges" {
            n198 = local read "_InterfaceFolderSuffix"() -> (w375:string)
            n199 = call <resource>:"BaseProvider_IniFileSettings.vi"() -> ("IniFileSettings"=w373:T20)  [unwired: 18 in, 1 out]
            n200 = Bundle By Name(cluster=w373, "InterfaceFolderSuffix"=w375) -> (w374:T20)
            n201 = Not Equal?(x=w374, y=w373) -> (x != y?=w372:bool)
            n202 = case shown="True" w372 {
              tunnel: w374 -> [_ w379]
              frame False {
              }
              frame True {
                n203 = call <resource>:"BaseProvider_IniFileSettings.vi"("IniFileSettings"=w379, "Action"=enum16{"Read", "Load", "Save"}."Save") -> ()  [unwired: 16 in, 2 out]
              }
            }
          }
          frame "Error", "Exit", Default {
          }
        }
      }
      n204 = call <resource>:"GDSString_AddStatesToQueue.vi"() -> ()  [unwired: 15 in, 1 out]
    }
    frame Error {
    }
  }
  "Reference out" <- w45
  "error out" <- w47
  n205 = call <resource>:"CommonVIs_ClassIconSelection.vi"("IconsToShow(All)"=CommonVIs_ClassIconSelection_Action."Only Interface", "Icon"=w22, "Messages(Stop or Empty string will stop this VI)"=w3, "IconSelection"=w21) -> ()  [unwired: 8 in]
  n206 = call <resource>:"GDSString_PlaceHolderText.vi"("BooleanUserEventToStopPlaceHolderVI"=w3, "PlaceholderText"="Interface name filter" ("InterfaceFilter"), "PlaceholderTextFont(Grey,Italic)"=T10 {"Font Name"="", "Size"=0, "Bold"=FALSE, "Italic"=TRUE, "Underline"=FALSE, "Strikeout"=FALSE, "Color"=10329501}, "NormalTextFont(Black)"=T10 {"Font Name"="", "Size"=0, "Bold"=FALSE, "Italic"=FALSE, "Underline"=FALSE, "Strikeout"=FALSE, "Color"=0}, "PlaceholderStringRef"=w7) -> ()  [unwired: 6 in, 1 out]
  n207 = Generate User Event(user event=w19, event data cluster="Stop" ("Stop")) -> (user event out=w20:refnum<user-event>)  [unwired: 2 in, 1 out]
  n208 = Destroy User Event(user event=w20) -> ()  [unwired: 1 in, 1 out]
  n209 = control-ref of="Wire Style"() -> (w2:refnum<vi>)
  n210 = control-ref of="WireSelectionList"() -> (w1:refnum<vi>)
  n211 = call <resource>:"CommonVIs_ClassWireSelection.vi"("Offset(-300,0)"=T9 {"Left"=-115, "Top"=18}, "SelectedWireStyle"=w2, "Messages(Stop or Empty string will stop this VI)"=w3, "WireSelectionList"=w1) -> ()  [unwired: 7 in, 1 out]
  n212 = stacked-sequence {
    tunnel: w43 -> [w392]
    tunnel: [w400] -> w42
    tunnel: [w399] -> w41
    tunnel: [w398] -> w40
    tunnel: [w397] -> w39
    tunnel: [w396] -> _
    tunnel: w16 -> [w393]
    tunnel: w38 -> [_]
    tunnel: [w391] -> w37
    tunnel: [w389] -> w12
    tunnel: [T8 {"InterfacePath"=[], "CreateMethods"=FALSE, "MethodsPerInterface(Empty=>All)"=[]} ("ParentInterfaces")] -> w11
    frame #0 {
      n213 = Unbundle By Name(w392) -> ("Cancel"=w400:bool, "DeriveFromClassRef"=w395:refnum<vi>)
      n214 = local read "_InterfaceFolder"() -> (w399:path)
      n215 = local read "_InterfaceName"() -> (w398:string)
      n216 = local read "_InterfaceFolderSuffix"() -> (w391:string)
      n217 = local read "_ClassDescription"() -> (w397:string)
      n218 = Not Equal?(x=w395, y=w393) -> (x != y?=w394:bool)
      n219 = case shown="True" w394 {
        tunnel: [_ w407] -> w396
        tunnel: w395 -> [_ w406]
        frame False {
        }
        frame True {
          n220 = Close Reference(reference=w406) -> (error out=w407:errorcluster)  [unwired: 1 in]
        }
      }
      n221 = for {
        tunnel: "Methods" -> [w405] mode=indexing
        tunnel: [w401] -> w389 mode=indexing
        n222 = Index Array(array=w405) -> (element #1=w403:string, element #2=w402:string)  [unwired: 2 in]
        n223 = Bundle By Name(cluster=T4 {"Name"="", "Description"="", "MethodsArgumentsIn"=[], "MethodsArgumentsOut"=[]} ("MethodToCreate"), "Name"=w403, "Description"=w402) -> (w401:T4)
      }
    }
  }
  "Cancelled" <- w42
  n224 = Bundle By Name(cluster=T3 {"InterfaceName"="", "InterfaceFolder"=path "", "InterfaceDescription"="", "FolderSuffix"="", "MethodsToCreate"=[], "ParentInterfaces"={"InterfacePath"=[], "CreateMethods"=FALSE, "MethodsPerInterface(Empty=>All)"=[]}} ("CreateInterfaceData"), "InterfaceFolder"=w41, "InterfaceName"=w40, "InterfaceDescription"=w39, "FolderSuffix"=w37, "MethodsToCreate"=w12, "ParentInterfaces"=w11) -> (→"CreateInterfaceData":T3)
